vi "Refine Corner Locations.vi"(5 "Zero Zone Size (Default: -1 x -1)":T1={"Width"=-1, "Height"=-1}, 6 "Termination Criteria (Default: Default Criteria)":refnum<class "Termination Criteria.lvclass">, 7 "Window Size (Default: 11 x 11)":T1={"Width"=11, "Height"=11}, 8 "error in (no error)":errorcluster, 10 "Points in":T2[](array[typedef]), 11 "Greyscale Image":refnum<data-value>) -> (0 "error out":errorcluster, 2 "Points out":T2[](array[typedef]), 3 "Greyscale Image (Duplicate)":refnum<data-value>)   [LabVIEW 2020, in "g_ar_toolkit.camera_calibration.lvlib"]
uses:
  g_ar_toolkit.camera_calibration.lvlib
  g_ar_toolkit.common/Image Point (Float).ctl
  g_ar_toolkit.common/Termination Criteria/Termination Criteria.lvclass
  g_ar_toolkit.common/Window Size (Integer).ctl
  bin/g_ar_toolkit.1.32.dll
  g_ar_toolkit.common/g_ar_toolkit.common.lvlib
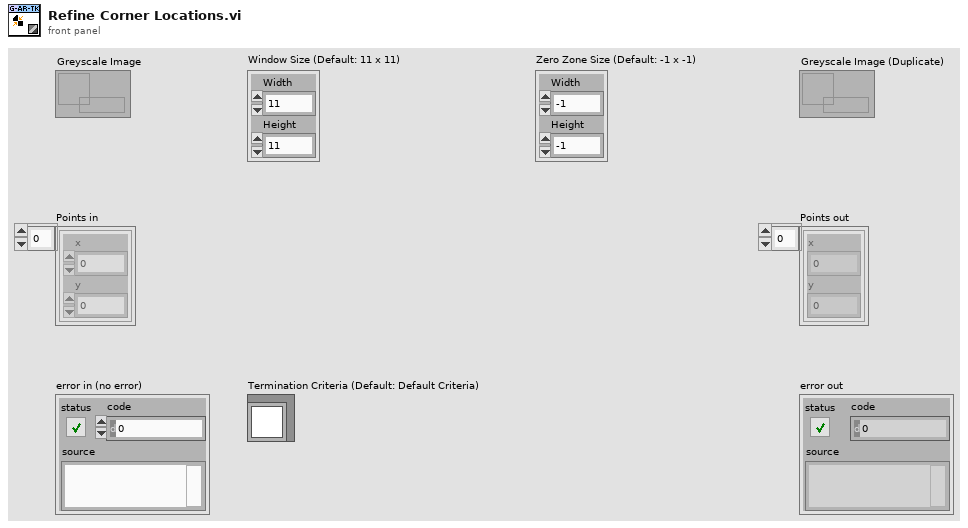
[diagram p1: front panel]
types:
  T1 = typedef "g_ar_toolkit.common.lvlib/Window Size (Integer).ctl" = cluster{"Width":i32, "Height":i32}
  T2 = typedef "g_ar_toolkit.common.lvlib/Image Point (Float).ctl" = cluster{"x":dbl, "y":dbl}
  T3 = typedef "g_ar_toolkit.common.lvlib/Termination Criteria.lvclass/Termination Criteria Values.ctl" = cluster{"Epsilon":dbl, "Iterations":i32}
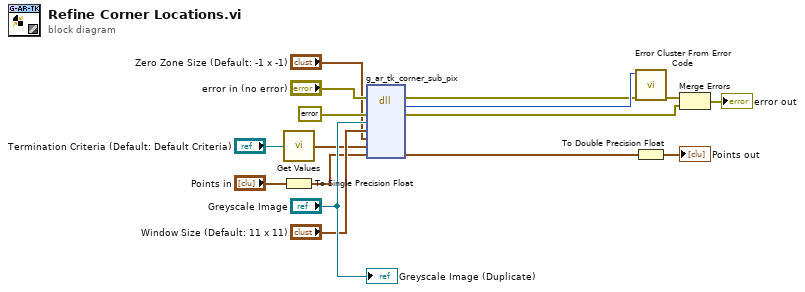
[diagram p0: block diagram]
diagram:
  n1 = call "Get Values.vi"("Termination Criteria in"="Termination Criteria (Default: Default Criteria)") -> ("Term Criteria"=w5:T3)
  n2 = To Single Precision Float(number="Points in") -> (single precision float=w3:cluster{"x":sgl, "y":sgl}[])
  n3 = dll-call lib="C:/serenial/libraries/g-augmented-reality-toolkit/LabVIEW/bin/g_ar_toolkit.1.*.*" fn="g_ar_tk_corner_sub_pix" ("g_ar_toolkit.*.*:g_ar_tk_image_draw_line")(error in="error in (no error)", "error_cluster"=errorcluster {"status"=FALSE, "code"=0, "source"=""} ("error constant"), "EDVR src"="Greyscale Image", "Window Size"="Window Size (Default: 11 x 11)", "Zero Zone"="Zero Zone Size (Default: -1 x -1)", "Termination Criteria"=w5, "Points"=w3) -> (error out=w12:errorcluster, "MgErr"=w13:i32, "error_cluster"=w16:errorcluster, "Points"=w2:cluster{"x":sgl, "y":sgl}[])  [unwired: 6 in, 1 out]
  n4 = call <vilib>:"Error Cluster From Error Code.vi"("error in (no error)"=w12, "error code (0)"=w13) -> ("error out"=w14:errorcluster)  [unwired: 7 in]
  n5 = To Double Precision Float(number=w2) -> (double precision float=→"Points out":cluster{"x":dbl, "y":dbl}[])
  n6 = Merge Errors(w14, w16) -> (→"error out":errorcluster)
  "Greyscale Image (Duplicate)" <- "Greyscale Image"
